vi "GenerateAttachablePosition_Pawn.vi"(1 "LastMovePiece":cluster{"Row":i32, "Column":i32, "IsMove":bool}, 2 "Black/White (T/F)":bool, 3 "pieceIndex":i32, 4 "Board":i32[][](array[numeric])=[[-3, -5, -4, -1, -2, -4, -5, -3], [-6, -6, -6, -6, -6, -6, -6, -6], [0, 0, 0, 0, 0, 0, 0, 0], [0, 0, 0, 0, 0, 0, 0, 0], [0, 0, 0, 0, 0, 0, 0, 0], [0, 0, 0, 0, 0, 0, 0, 0], [6, 6, 6, 6, 6, 6, 6, 6], [3, 5, 4, 1, 2, 4, 5, 3]]) -> (0 "AttachablePosition":bool[][](array[boolean]))   [LabVIEW 2014]
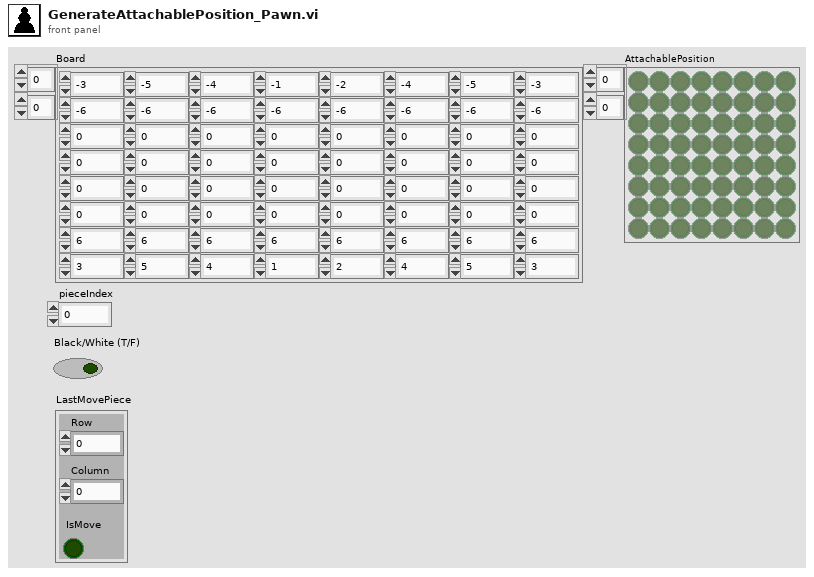
[diagram p1: front panel]
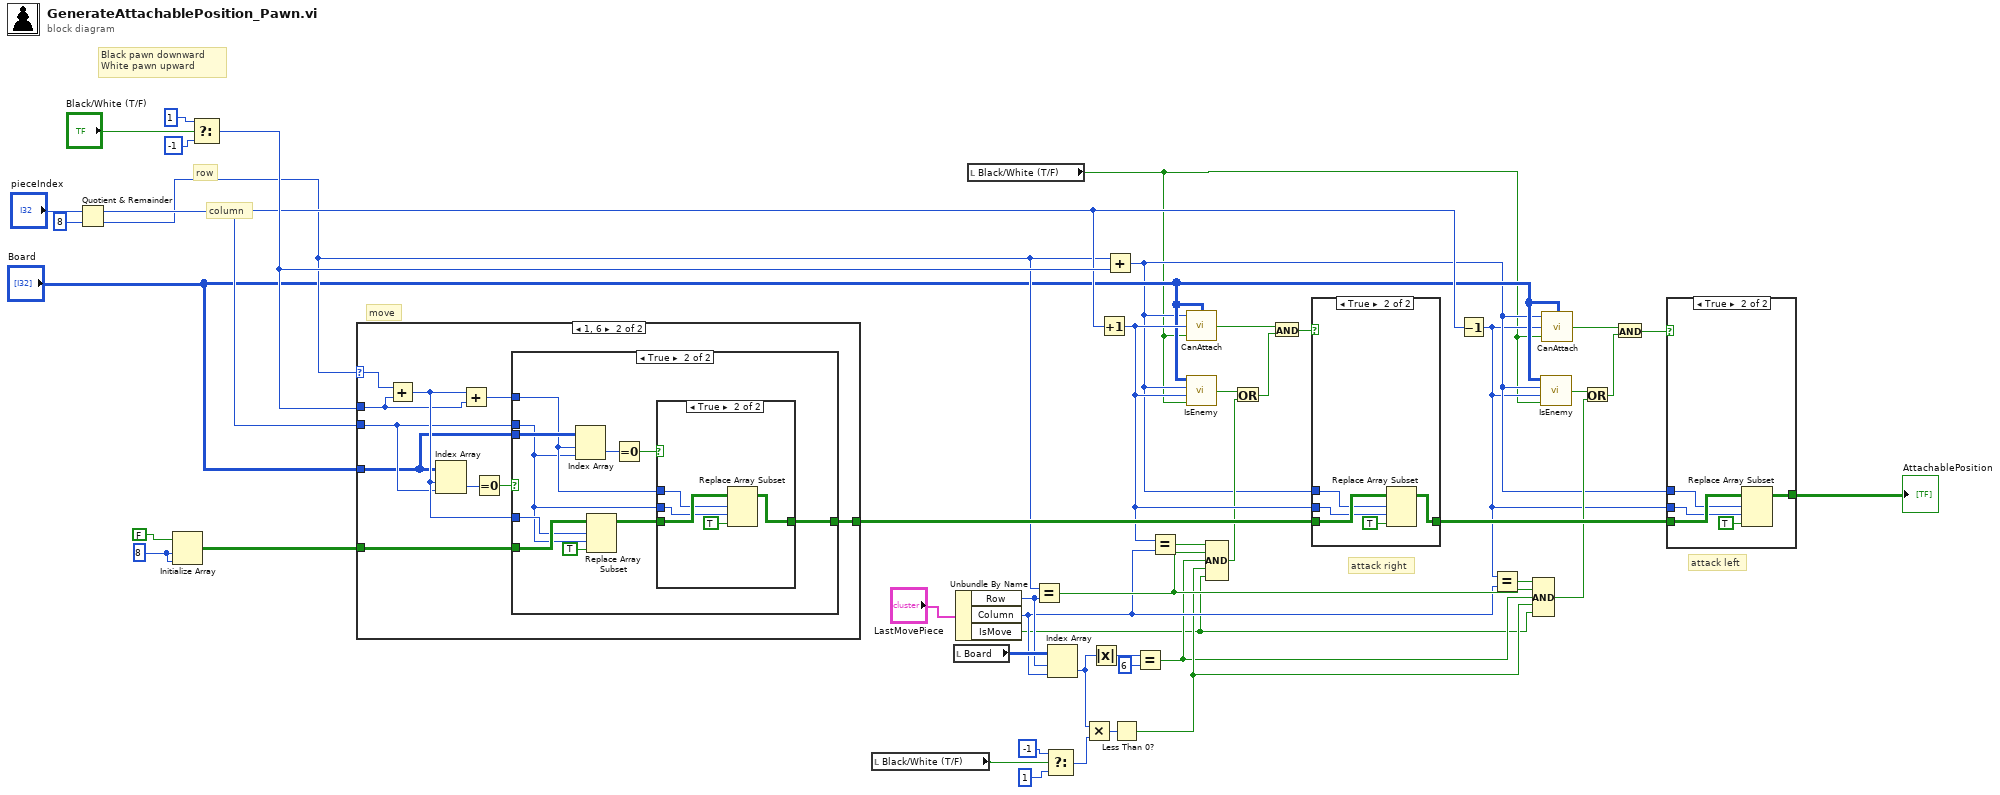
[diagram p0: block diagram]
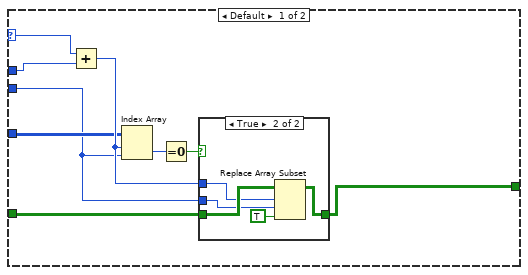
[diagram p4: hidden frame]
diagram:
  w45 = 8 ("dimension size")
  # "attack left"
  # "attack right"
  # "move"
  # "Black pawn downward\nWhite pawn upward"
  # "column"
  # "row"
  n1 = Quotient & Remainder(x="pieceIndex", y=8) -> (x-y*floor(x/y)=w38:i32, floor(x/y)=w33:i32)
  n2 = Initialize Array(FALSE, w45, w45) -> (w40:bool[][])
  n3 = Select(t=1, s="Black/White (T/F)", f=-1) -> (s? t:f=w39:i32)
  n4 = case shown="1, 6" w33 {
    selector: w33 -> [w48 w72]
    tunnel: w39 -> [w51 w66]
    tunnel: w40 -> [w50 w69]
    tunnel: w38 -> [w52 w64]
    tunnel: "Board" -> [w53 w63]
    tunnel: [w49 w68] -> w37
    frame Default {
      n5 = Add(x=w48, y=w51) -> (x+y=w54:i32)
      n6 = Index Array(array=w53, index (row)=w54, index (col)=w52) -> (element=w56:i32)
      n7 = Equal To 0?(x=w56) -> (x = 0?=w55:bool)
      n8 = case shown="True" w55 {
        tunnel: w50 -> [w57 w62]
        tunnel: w54 -> [_ w61]
        tunnel: w52 -> [_ w60]
        tunnel: [w57 w58] -> w49
        frame False {
        }
        frame True {
          n9 = Replace Array Subset(array=w62, new element=TRUE ("new element/subarray"), index (row)=w61, index (col)=w60) -> (w58:bool[][])
        }
      }
    }
    frame 1, 6 {
      n10 = Add(x=w72, y=w66) -> (x+y=w67:i32)
      n11 = Index Array(array=w63, index (row)=w67, index (col)=w64) -> (element=w71:i32)
      n12 = Add(x=w67, y=w66) -> (x+y=w65:i32)
      n13 = Equal To 0?(x=w71) -> (x = 0?=w70:bool)
      n14 = case shown="True" w70 {
        tunnel: w69 -> [w73 w83]
        tunnel: w67 -> [_ w82]
        tunnel: [w73 w79] -> w68
        tunnel: w65 -> [_ w75]
        tunnel: w64 -> [_ w74]
        tunnel: w63 -> [_ w77]
        frame False {
        }
        frame True {
          n15 = Index Array(array=w77, index (row)=w75, index (col)=w74) -> (element=w78:i32)
          n16 = Replace Array Subset(array=w83, new element=TRUE ("new element/subarray"), index (row)=w82, index (col)=w74) -> (w80:bool[][])
          n17 = Equal To 0?(x=w78) -> (x = 0?=w76:bool)
          n18 = case shown="True" w76 {
            tunnel: w80 -> [w84 w89]
            tunnel: w75 -> [_ w88]
            tunnel: w74 -> [_ w87]
            tunnel: [w84 w85] -> w79
            frame False {
            }
            frame True {
              n19 = Replace Array Subset(array=w89, new element=TRUE ("new element/subarray"), index (row)=w88, index (col)=w87) -> (w85:bool[][])
            }
          }
        }
      }
    }
  }
  n20 = local read "Black/White (T/F)"() -> (w22:bool)
  n21 = local read "Board"() -> (w27:i32[][])
  n22 = Unbundle By Name("LastMovePiece") -> ("Row"=w26:i32, "Column"=w25:i32, "IsMove"=w1:bool)
  n23 = local read "Black/White (T/F)"() -> (w2:bool)
  n24 = Equal?(x=w33, y=w26) -> (x = y?=w29:bool)
  n25 = Select(t=-1, s=w22, f=1) -> (s? t:f=w21:i32)
  n26 = Index Array(array=w27, index (row)=w26, index (col)=w25) -> (element=w17:i32)
  n27 = Multiply(x=w17, y=w21) -> (x*y=w20:i32)
  n28 = Absolute Value(x=w17) -> (abs(x)=w15:i32)
  n29 = Increment(x=w38) -> (x+1=w12:i32)
  n30 = Add(x=w33, y=w39) -> (x+y=w4:i32)
  n31 = Less Than 0?(x=w20) -> (x < 0?=w16:bool)
  n32 = Equal?(x=w15, y=6) -> (x = y?=w13:bool)
  n33 = Equal?(x=w12, y=w25) -> (x = y?=w32:bool)
  n34 = call "CanAttach.vi"("Board"="Board", "Black/White Turn (T/F)"=w2, "Column"=w12, "Row"=w4) -> ("Boolean"=w18:bool)
  n35 = call "IsEnemy.vi"("Black/White Turn (T/F)"=w2, "Column"=w12, "Row"=w4, "Board"="Board") -> ("Boolean"=w10:bool)
  n36 = Compound Arithmetic op=AND(w32, w29, w13, w16, w1) -> (w9:bool)
  n37 = Or(x=w10, y=w9) -> (x .or. y?=w11:bool)
  n38 = And(x=w18, y=w11) -> (x .and. y?=w19:bool)
  n39 = case shown="True" w19 {
    tunnel: w37 -> [w90 w95]
    tunnel: w4 -> [_ w94]
    tunnel: w12 -> [_ w93]
    tunnel: [w90 w91] -> w36
    frame False {
    }
    frame True {
      n40 = Replace Array Subset(array=w95, new element=TRUE ("new element/subarray"), index (row)=w94, index (col)=w93) -> (w91:bool[][])
    }
  }
  n41 = Decrement(x=w38) -> (x-1=w3:i32)
  n42 = Equal?(x=w3, y=w25) -> (x = y?=w30:bool)
  n43 = Compound Arithmetic op=AND(w30, w29, w13, w16, w1) -> (w7:bool)
  n44 = call "IsEnemy.vi"("Black/White Turn (T/F)"=w2, "Column"=w3, "Row"=w4, "Board"="Board") -> ("Boolean"=w6:bool)
  n45 = call "CanAttach.vi"("Board"="Board", "Black/White Turn (T/F)"=w2, "Column"=w3, "Row"=w4) -> ("Boolean"=w28:bool)
  n46 = Or(x=w6, y=w7) -> (x .or. y?=w8:bool)
  n47 = And(x=w28, y=w8) -> (x .and. y?=w31:bool)
  n48 = case shown="True" w31 {
    tunnel: w36 -> [w96 w101]
    tunnel: w4 -> [_ w100]
    tunnel: w3 -> [_ w99]
    tunnel: [w96 w97] -> w35
    frame False {
    }
    frame True {
      n49 = Replace Array Subset(array=w101, new element=TRUE ("new element/subarray"), index (row)=w100, index (col)=w99) -> (w97:bool[][])
    }
  }
  "AttachablePosition" <- w35
